vi "Configure Instruments.vi"(6 "Magnet":T2, 7 "Ammeter":T3=enum."648X", 8 "error in (no error)":errorcluster, 9 "Voltmeter":T5=enum."2182A", 10 "Switch":T1, 11 "Current Source":T4=enum."26XX") -> (0 "error out":errorcluster)   [LabVIEW 2016, in "Hall Effect Library.lvlib"]
uses:
  Hall Effect Library.lvlib
  Controls/Voltmeters.ctl
  Controls/I-Sources.ctl
  Controls/Ammeters.ctl
  Controls/Magnets.ctl
  Controls/Switches.ctl
  Private/Global Variables/Instruments.vi
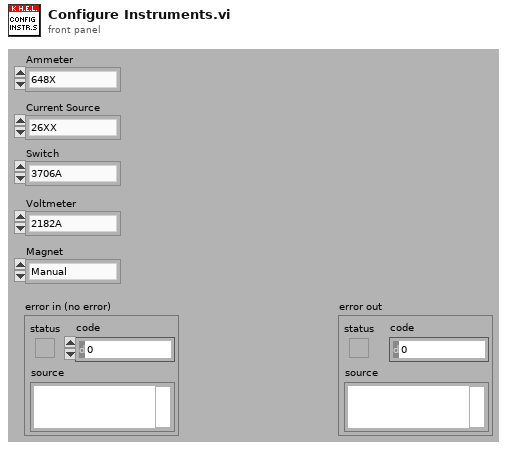
[diagram p1: front panel]
types:
  T1 = typedef "Hall Effect Library.lvlib/Switches.ctl" = enum16{"3706A"}
  T2 = typedef "Hall Effect Library.lvlib/Magnets.ctl" = enum16{"Manual"}
  T3 = typedef "Hall Effect Library.lvlib/Ammeters.ctl" = enum16{"None", "648X"}
  T4 = typedef "Hall Effect Library.lvlib/I-Sources.ctl" = enum16{"622X", "26XX"}
  T5 = typedef "Hall Effect Library.lvlib/Voltmeters.ctl" = enum16{"2000", "2182A", "3706A"}
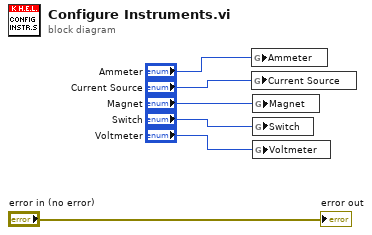
[diagram p0: block diagram]
diagram:
  n1 = global write "Instruments.vi" "Ammeter"("Ammeter") -> ()
  n2 = global write "Instruments.vi" "Current Source"("Current Source") -> ()
  n3 = global write "Instruments.vi" "Magnet"("Magnet") -> ()
  n4 = global write "Instruments.vi" "Switch"("Switch") -> ()
  n5 = global write "Instruments.vi" "Voltmeter"("Voltmeter") -> ()
  "error out" <- "error in (no error)"
